vi "DAQmx TC01.vi"() -> (0 "Temperature data":dbl)   [LabVIEW 2023]
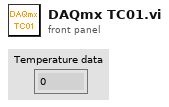
[diagram p1: front panel]
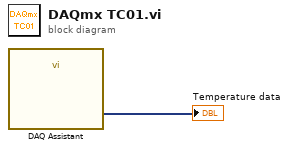
[diagram p0: block diagram]
diagram:
  n1 = call "DAQ Assistant"() -> ("data"=→"Temperature data":dynamicdata)  [unwired: 17 in, 2 out]
